vi "DOWaveAction.vi"(6 "Slot":T1, 7 "循环次数":u32=50, 8 "error in":errorcluster, 9 "后段延时":dbl=10.0, 10 "前段延时":dbl=20.0, 11 "CH":string) -> (0 "error out":errorcluster)   [LabVIEW 2013]
uses:
  SystemCode/SysControl/Slot.ctl
  <vilib>/DAQmx/write.llb/DAQmx Write (Digital Bool 1Line 1Point).vi
  <vilib>/DAQmx/read.llb/DAQmx Read (Digital Bool 1Line 1Point).vi
  SourceCode/GlobalValue.vi
  Xmodem_2_FileReceive/FileGolbalPara.vi
  <vilib>/DAQmx/create/channels.llb/DAQmx Create Channel (DO-Digital Output).vi
  <vilib>/DAQmx/miscellaneous.llb/DAQmx Fill In Error Info.vi
panel:
  out "数值":i32
  out "波形图表":i16(graph)
  in  "Debug":bool
  in  "State":string="1"
  out "DO status":bool
  out "State":bool
  out "Line/port":tag="PCI-6229/port0/line0:1"
  in  "Enum":enum16{"Set", "Get", "Initialize"}(ring)
  # "CylinderCtrl"
  # "B+"
  # "ACC"
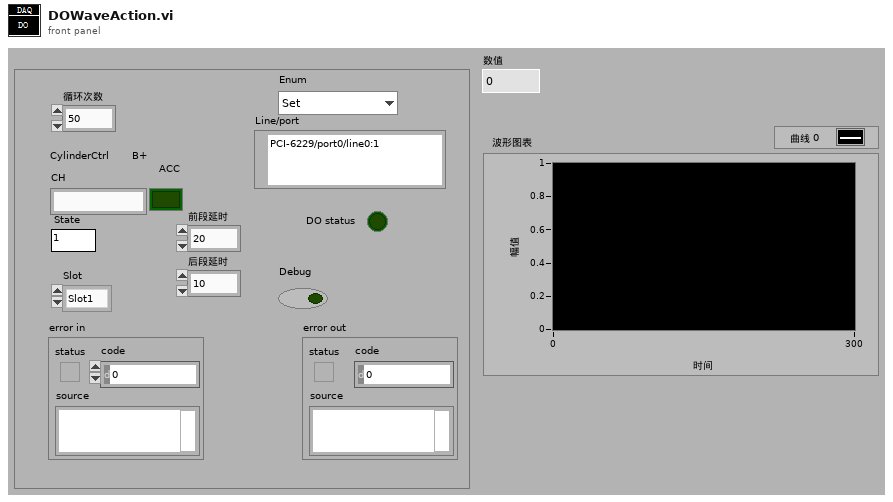
[diagram p1: front panel]
types:
  T1 = typedef "Slot.ctl" = enum16{"Slot1", "Slot2", "Slot3", "Slot4"}
  T2 = typedef "DAQConfig.ctl" = cluster{"DIO":string[][], "AO":string[][], "AI":string[][]}
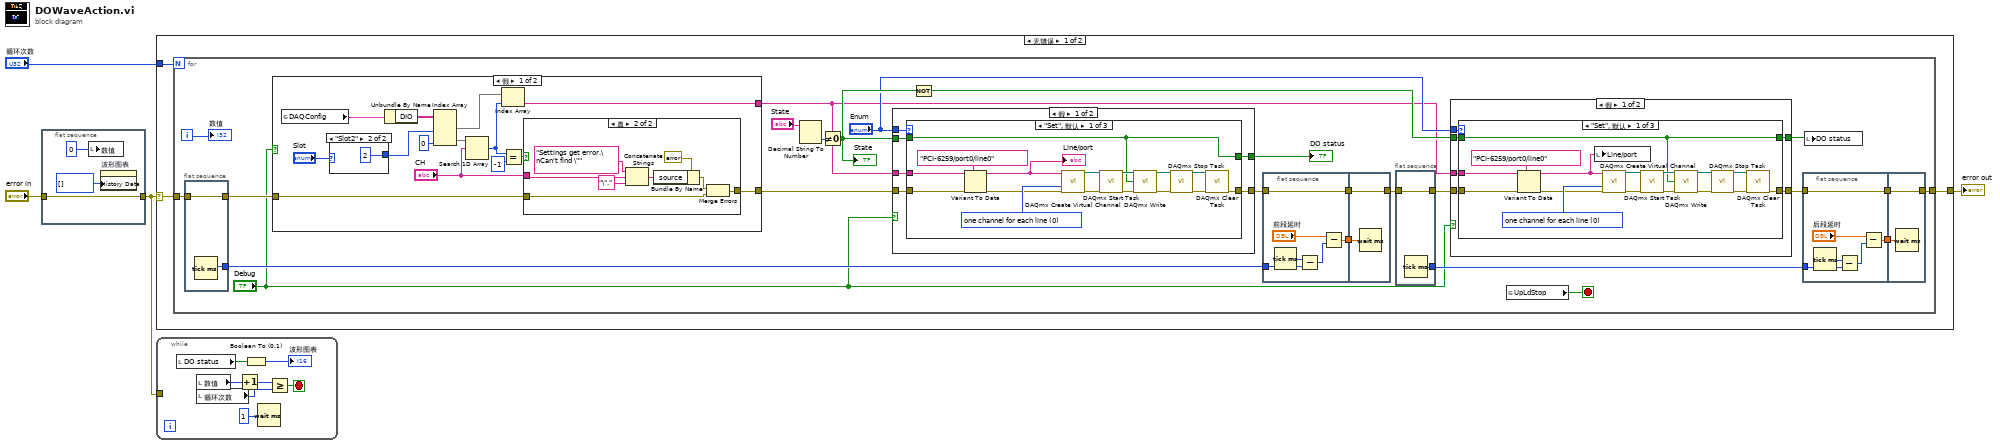
[diagram p0: block diagram]
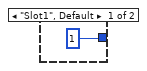
[diagram p2: hidden frame]
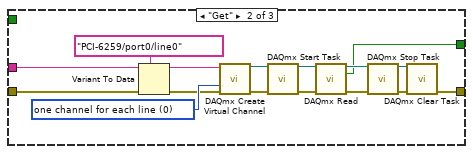
[diagram p5: hidden frame]
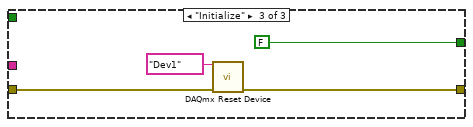
[diagram p6: hidden frame]
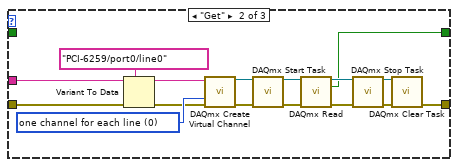
[diagram p8: hidden frame]
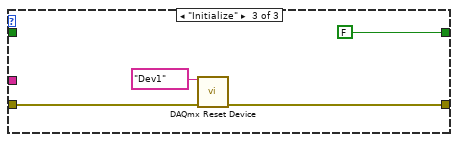
[diagram p9: hidden frame]
diagram:
  n1 = flat-sequence {
    tunnel: [w7] -> w1
    tunnel: "error in" -> [w7]
    frame #0 {
      n2 = local write "数值"(0 ("数值")) -> ()
      n3 = property on="波形图表" class="WFChart (严格)"("History Data"=i16[] [] ("历史数据")) -> ()  [unwired: 2 in, 2 out]
    }
  }
  n4 = case shown="无错误" w1 {
    selector: w1 -> [w10 w170]
    tunnel: [w9 w170] -> w4
    tunnel: "循环次数" -> [w8 _]
    frame No Error {
      n5 = for {
        N: w8 -> [_]
        tunnel: w10 -> [w27]
        tunnel: [w17] -> w9
        i -> [w12]
        stop <- w11 stop-if-true
        n6 = flat-sequence {
          tunnel: [w169] -> w28
          tunnel: w27 -> [w169]
          tunnel: [w168] -> w25
          frame #0 {
            n7 = Tick Count (ms)() -> (millisecond timer value=w168:u32)
          }
        }
        n8 = case shown="假" "Debug" {
          tunnel: [w44 w61] -> w31
          tunnel: w28 -> [w37 w61]
          tunnel: [w36 _] -> w21
          frame False {
            n9 = global read "GlobalValue.vi" "DAQConfig"() -> (w38:T2)
            n10 = case shown="\"Slot2\"" "Slot" {
              tunnel: [1 ("索引 (行)") 2 ("索引 (行)")] -> w39
              frame "Slot1", Default {
              }
              frame "Slot2" {
              }
            }
            n11 = Unbundle By Name(w38) -> ("DIO"=w49:string[][])
            n12 = Index Array(array=w49, index (col) #1=w39, index (col) #2=0 ("索引 (列)")) -> (element #1=w42:string[], element #2=w41:string[])  [unwired: 2 in]
            n13 = Search 1D Array(1D array=w41, element="CH") -> (index of element=w47:i32)  [unwired: 1 in]
            n14 = Index Array(array=w42, index=w47) -> (element=w36:string)
            n15 = Equal?(x=w47, y=-1) -> (x = y?=w45:bool)
            n16 = case shown="真" w45 {
              tunnel: "CH" -> [_ w56]
              tunnel: w37 -> [w52 w55]
              tunnel: [w52 w54] -> w44
              frame False {
              }
              frame True {
                n17 = Concatenate Strings("Settings get error.\nCan't find \"" ("message"), w56, "\"." ("string")) -> (w59:string)
                n18 = Bundle By Name(cluster=errorcluster {"status"=TRUE, "code"=5000, "source"=""} ("error in 1 (no error)"), "source"=w59) -> (w58:errorcluster)
                n19 = Merge Errors(w58, w55) -> (w54:errorcluster)
              }
            }
          }
          frame True {
          }
        }
        n20 = Decimal String To Number(string="State") -> (number=w30:i32)  [unwired: 2 in, 1 out]
        n21 = Not Equal To 0?(x=w30) -> (x != 0?=w24:bool)
        "State" <- w24
        n22 = case shown="假" "Debug" {
          tunnel: w31 -> [w67 w104]
          tunnel: [w66 w104] -> w26
          tunnel: w24 -> [w65 w105]
          tunnel: "Enum" -> [w64 _]
          tunnel: w21 -> [w63 _]
          tunnel: [w62 w105] -> w15
          frame False {
            n23 = case shown="\"Set\", 默认" w64 {
              tunnel: w67 -> [w69 w84 w103]
              tunnel: [w77 w93 w102] -> w66
              tunnel: [w68 w86 FALSE ("data")] -> w62
              tunnel: w63 -> [w70 w85 _]
              tunnel: w65 -> [w68 _ _]
              frame "Set", Default {
                w72 = 0 items=["one channel for each line", "one channel for all lines"] ("line grouping")
                n24 = Variant To Data(error in=w69, type=tag "PCI-6259/port0/line0" ("lines"), Variant=w70) -> (data=w75:tag, error out=w71:errorcluster)
                "Line/port" <- w75
                n25 = call-poly <vilib>:"DAQmx Create Virtual Channel.vi"("lines"=w75, "line grouping"=w72, "error in"=w71) -> ("task out"=w83:refnum<k21>, "error out"=w82:errorcluster)  [unwired: 11 in]
                n26 = call <vilib>:"DAQmx Start Task.vi"("task/channels in"=w83, "error in"=w82) -> ("task out"=w81:refnum<k21>, "error out"=w80:errorcluster)  [unwired: 12 in]
                n27 = call-poly <vilib>:"DAQmx Write.vi"("task/channels in"=w81, "data"=w68, "error in"=w80) -> ("task out"=w74:refnum<k21>, "error out"=w73:errorcluster)  [unwired: 10 in, 1 out]
                n28 = call <vilib>:"DAQmx Stop Task.vi"("task/channels in"=w74, "error in"=w73) -> ("task out"=w79:refnum<k21>, "error out"=w78:errorcluster)  [unwired: 12 in]
                n29 = call <vilib>:"DAQmx Clear Task.vi"("task in"=w79, "error in"=w78) -> ("error out"=w77:errorcluster)  [unwired: 13 in]
              }
              frame "Get" {
                w92 = 0 items=["one channel for each line", "one channel for all lines"] ("line grouping")
                n30 = Variant To Data(error in=w84, type=tag "PCI-6259/port0/line0" ("lines"), Variant=w85) -> (data=w90:tag, error out=w89:errorcluster)
                n31 = call-poly <vilib>:"DAQmx Create Virtual Channel.vi"("lines"=w90, "line grouping"=w92, "error in"=w89) -> ("task out"=w99:refnum<k21>, "error out"=w98:errorcluster)  [unwired: 11 in]
                n32 = call <vilib>:"DAQmx Start Task.vi"("task/channels in"=w99, "error in"=w98) -> ("task out"=w97:refnum<k21>, "error out"=w96:errorcluster)  [unwired: 12 in]
                n33 = call-poly <vilib>:"DAQmx Read.vi"("task/channels in"=w97, "error in"=w96) -> ("task out"=w88:refnum<k21>, "data"=w86:bool, "error out"=w87:errorcluster)  [unwired: 11 in]
                n34 = call <vilib>:"DAQmx Stop Task.vi"("task/channels in"=w88, "error in"=w87) -> ("task out"=w95:refnum<k21>, "error out"=w94:errorcluster)  [unwired: 12 in]
                n35 = call <vilib>:"DAQmx Clear Task.vi"("task in"=w95, "error in"=w94) -> ("error out"=w93:errorcluster)  [unwired: 13 in]
              }
              frame "Initialize" {
                n36 = call <vilib>:"DAQmx Reset Device.vi"("device in"=tag "Dev1", "error in"=w103) -> ("error out"=w102:errorcluster)  [unwired: 13 in]
              }
            }
          }
          frame True {
          }
        }
        "DO status" <- w15
        n37 = Not(x=w24) -> (.not. x?=w23:bool)
        n38 = flat-sequence {
          tunnel: w26 -> [w165]
          tunnel: [w165] -> w35
          tunnel: w25 -> [w164]
          tunnel: [w160] -> w34
          tunnel: [w167] -> w20
          tunnel: w35 -> [w167]
          tunnel: w34 -> [w166]
          frame #0 {
            n39 = Tick Count (ms)() -> (millisecond timer value=w163:u32)
            n40 = Subtract(x=w163, y=w164) -> (x-y=w162:u32)
            n41 = Subtract(x="前段延时", y=w162) -> (x-y=w160:dbl)
          }
          frame #1 {
            n42 = Wait (ms)(milliseconds to wait=w166) -> ()  [unwired: 1 out]
          }
        }
        n43 = flat-sequence {
          tunnel: w20 -> [w159]
          tunnel: [w159] -> w19
          tunnel: [w158] -> w16
          frame #0 {
            n44 = Tick Count (ms)() -> (millisecond timer value=w158:u32)
          }
        }
        n45 = case shown="假" "Debug" {
          tunnel: w23 -> [w111 w149]
          tunnel: "Enum" -> [w110 _]
          tunnel: w21 -> [w109 _]
          tunnel: w19 -> [w108 w148]
          tunnel: [w107 w148] -> w18
          tunnel: [w106 w149] -> w14
          frame False {
            n46 = case shown="\"Set\", 默认" w110 {
              tunnel: w108 -> [w114 w128 w147]
              tunnel: [w121 w137 w146] -> w107
              tunnel: [w113 w130 FALSE ("data")] -> w106
              tunnel: w109 -> [w115 w129 _]
              tunnel: w111 -> [w113 _ _]
              frame "Set", Default {
                w117 = 0 items=["one channel for each line", "one channel for all lines"] ("line grouping")
                n47 = Variant To Data(error in=w114, type=tag "PCI-6259/port0/line0" ("lines"), Variant=w115) -> (data=w112:tag, error out=w116:errorcluster)
                n48 = local write "Line/port"(w112) -> ()
                n49 = call-poly <vilib>:"DAQmx Create Virtual Channel.vi"("lines"=w112, "line grouping"=w117, "error in"=w116) -> ("task out"=w127:refnum<k21>, "error out"=w126:errorcluster)  [unwired: 11 in]
                n50 = call <vilib>:"DAQmx Start Task.vi"("task/channels in"=w127, "error in"=w126) -> ("task out"=w125:refnum<k21>, "error out"=w124:errorcluster)  [unwired: 12 in]
                n51 = call-poly <vilib>:"DAQmx Write.vi"("task/channels in"=w125, "data"=w113, "error in"=w124) -> ("task out"=w119:refnum<k21>, "error out"=w118:errorcluster)  [unwired: 10 in, 1 out]
                n52 = call <vilib>:"DAQmx Stop Task.vi"("task/channels in"=w119, "error in"=w118) -> ("task out"=w123:refnum<k21>, "error out"=w122:errorcluster)  [unwired: 12 in]
                n53 = call <vilib>:"DAQmx Clear Task.vi"("task in"=w123, "error in"=w122) -> ("error out"=w121:errorcluster)  [unwired: 13 in]
              }
              frame "Get" {
                w136 = 0 items=["one channel for each line", "one channel for all lines"] ("line grouping")
                n54 = Variant To Data(error in=w128, type=tag "PCI-6259/port0/line0" ("lines"), Variant=w129) -> (data=w134:tag, error out=w133:errorcluster)
                n55 = call-poly <vilib>:"DAQmx Create Virtual Channel.vi"("lines"=w134, "line grouping"=w136, "error in"=w133) -> ("task out"=w143:refnum<k21>, "error out"=w142:errorcluster)  [unwired: 11 in]
                n56 = call <vilib>:"DAQmx Start Task.vi"("task/channels in"=w143, "error in"=w142) -> ("task out"=w141:refnum<k21>, "error out"=w140:errorcluster)  [unwired: 12 in]
                n57 = call-poly <vilib>:"DAQmx Read.vi"("task/channels in"=w141, "error in"=w140) -> ("task out"=w132:refnum<k21>, "data"=w130:bool, "error out"=w131:errorcluster)  [unwired: 11 in]
                n58 = call <vilib>:"DAQmx Stop Task.vi"("task/channels in"=w132, "error in"=w131) -> ("task out"=w139:refnum<k21>, "error out"=w138:errorcluster)  [unwired: 12 in]
                n59 = call <vilib>:"DAQmx Clear Task.vi"("task in"=w139, "error in"=w138) -> ("error out"=w137:errorcluster)  [unwired: 13 in]
              }
              frame "Initialize" {
                n60 = call <vilib>:"DAQmx Reset Device.vi"("device in"=tag "Dev1", "error in"=w147) -> ("error out"=w146:errorcluster)  [unwired: 13 in]
              }
            }
          }
          frame True {
          }
        }
        n61 = global read "FileGolbalPara.vi" "UpLdStop"() -> (w11:bool)
        n62 = flat-sequence {
          tunnel: w18 -> [w155]
          tunnel: [w155] -> w33
          tunnel: w16 -> [w154]
          tunnel: [w150] -> w32
          tunnel: [w157] -> w17
          tunnel: w33 -> [w157]
          tunnel: w32 -> [w156]
          frame #0 {
            n63 = Tick Count (ms)() -> (millisecond timer value=w153:u32)
            n64 = Subtract(x=w153, y=w154) -> (x-y=w152:u32)
            n65 = Subtract(x="后段延时", y=w152) -> (x-y=w150:dbl)
          }
          frame #1 {
            n66 = Wait (ms)(milliseconds to wait=w156) -> ()  [unwired: 1 out]
          }
        }
        n67 = local write "DO status"(w14) -> ()
        "数值" <- w12
      }
    }
    frame Error {
    }
  }
  "error out" <- w4
  n68 = while {
    tunnel: w1 -> [_]
    stop <- w172 stop-if-true
    n69 = local read "DO status"() -> (w176:bool)
    n70 = local read "数值"() -> (w174:i32)
    n71 = local read "循环次数"() -> (w173:u32)
    n72 = Increment(x=w174) -> (x+1=w171:i32)
    n73 = Boolean To (0,1)(Boolean=w176) -> (0, 1=→"波形图表":i16)
    n74 = Wait (ms)(milliseconds to wait=u32 1 ("等待时间（毫秒）")) -> ()  [unwired: 1 out]
    n75 = Greater Or Equal?(x=w171, y=w173) -> (x >= y?=w172:bool)
  }
